vi "Main test.vi"() -> ()   [LabVIEW 2021]
uses:
  Lib/Rigol DMM/Functions.ctl
  Lib/Rigol DMM/Trig sources.ctl
  Lib/Rigol DMM/Rigol DM3052.lvlib
panel:
  in  "Boolean":bool
  in  "milliseconds to wait":u32
  in  "Interval (100ms)":u32=100 min=8 max=2000 step=1
  in  "Source (auto)":T1
  out "value":dbl
  in  "Function":T2
  out "error out":errorcluster
  out "answer":string
  in  "PORT (GPIB)":refnum<visa-resource-name>="GPIB0::4::INSTR"
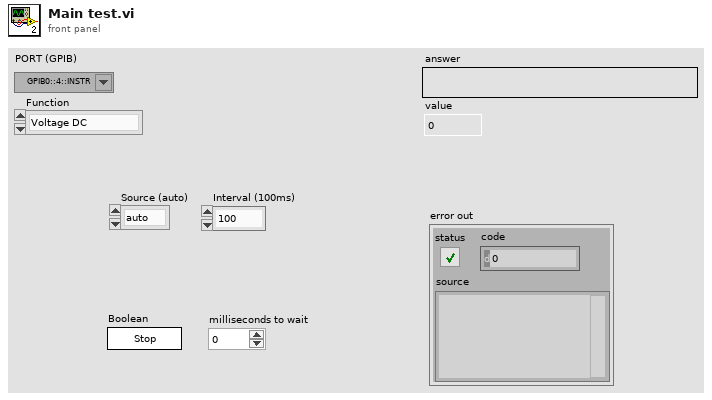
[diagram p1: front panel]
types:
  T1 = typedef "Rigol DM3052.lvlib/Trig sources.ctl" = enum16{"auto", "single", "ext"}
  T2 = typedef "Rigol DM3052.lvlib/Functions.ctl" = enum16{"Voltage DC", "Voltage AC", "Current DC", "Current AC", "Continuity", "Diode", "Resistance"}
  T3 = typedef "Rigol DM3052.lvlib/Reference.ctl" = cluster{"Device":refnum<visa-resource-name>, "Function":string, "delay":u32}
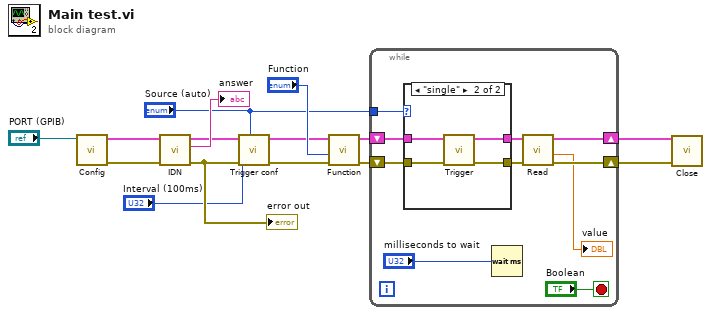
[diagram p0: block diagram]
diagram:
  n1 = call "Config.vi"("PORT (GPIB)"="PORT (GPIB)") -> ("error out"=w14:errorcluster, "Reference out"=w12:T3)  [unwired: 9 in]
  n2 = call "IDN.vi"("error in (no error)"=w14, "Reference in"=w12) -> ("error out"=w6:errorcluster, "answer"=→"answer":string, "Reference out"=w7:T3)  [unwired: 7 in]
  "error out" <- w6
  n3 = call "Trigger conf.vi"("Source (auto)"="Source (auto)", "error in (no error)"=w6, "Interval (100ms)"="Interval (100ms)", "Reference in"=w7) -> ("error out"=w5:errorcluster, "Reference out"=w4:T3)  [unwired: 5 in, 1 out]
  n4 = call "Function.vi"("error in (no error)"=w5, "Function"="Function", "Reference in"=w4) -> ("error out"=w10:errorcluster, "Reference out"=w2:T3)  [unwired: 6 in, 1 out]
  n5 = while {
    tunnel: "Source (auto)" -> [w18]
    shift-right: [w24] -> w9
    shift-left: w10 -> [w25]
    shift-right: [w23] -> w8
    shift-left: w2 -> [w20]
    stop <- "Boolean" stop-if-true
    n6 = case shown="\"single\"" w18 {
      tunnel: w25 -> [w26 w31]
      tunnel: [w26 w30] -> w21
      tunnel: w20 -> [w27 w29]
      tunnel: [w27 w28] -> w19
      frame "auto", Default {
      }
      frame "single" {
        n7 = call "Trigger.vi"("error in (no error)"=w31, "Reference in"=w29) -> ("error out"=w30:errorcluster, "Reference out"=w28:T3)  [unwired: 7 in, 1 out]
      }
    }
    n8 = Wait (ms)(milliseconds to wait="milliseconds to wait") -> ()  [unwired: 1 out]
    n9 = call "Read.vi"("error in (no error)"=w21, "Reference in"=w19) -> ("error out"=w24:errorcluster, "value"=→"value":dbl, "Reference out"=w23:T3)  [unwired: 6 in, 1 out]
  }
  n10 = call "Close.vi"("error in (no error)"=w9, "Reference in"=w8) -> ()  [unwired: 9 in, 1 out]
